vi "Simulated_AnalogOutput.vi"(10 "data":dbl, 11 "Device Name":tag) -> (0 "error out":errorcluster)   [LabVIEW 2023]
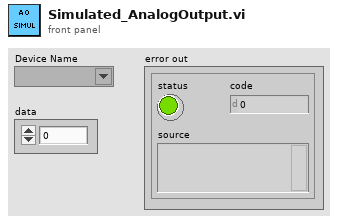
[diagram p1: front panel]
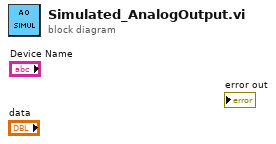
[diagram p0: block diagram]
diagram:
